vi "Brama_Sub_VI.vi"(6 "Enum in":T1(ring), 7 "Brama 1 - kto pierwszy":T5(ring), 9 "Brama 1":T4, 10 "reference in":refnum<vi>, 11 "Digital in":refnum<vi>) -> (2 "Enum out":T1(ring), 3 "Brama 2":T3)   [LabVIEW 2017]
uses:
  Str_Lam&Sil.ctl
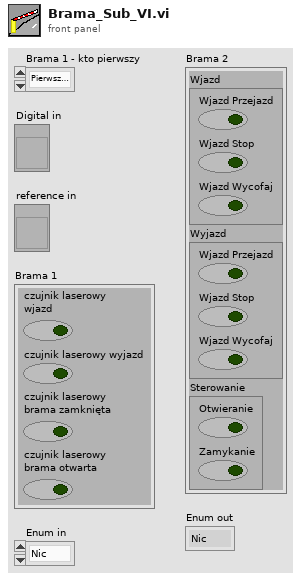
[diagram p1: front panel]
types:
  T1 = enum16{"Nic", "Otwieranie", "Otwarte", "Wjazd", "Wyjazd", "Zamykanie", "Wycofaj", "Blad"}
  T2 = typedef "Str_Lam&Sil.ctl" = bool
  T3 = cluster{"Wjazd":cluster{"Wjazd Przejazd":T2, "Wjazd Stop":bool, "Wjazd Wycofaj":bool}, "Wyjazd":cluster{"Wjazd Przejazd":bool, "Wjazd Stop":bool, "Wjazd Wycofaj":bool}, "Sterowanie":cluster{"Otwieranie":bool, "Zamykanie":bool}}
  T4 = cluster{"czujnik laserowy \nwjazd":bool, "czujnik laserowy wyjazd":bool, "czujnik laserowy \nbrama zamknięta":bool, "czujnik laserowy \nbrama otwarta":bool}
  T5 = enum16{"Pierwszy wjazd", "Nikt", "Pierwszy wyjazd"}
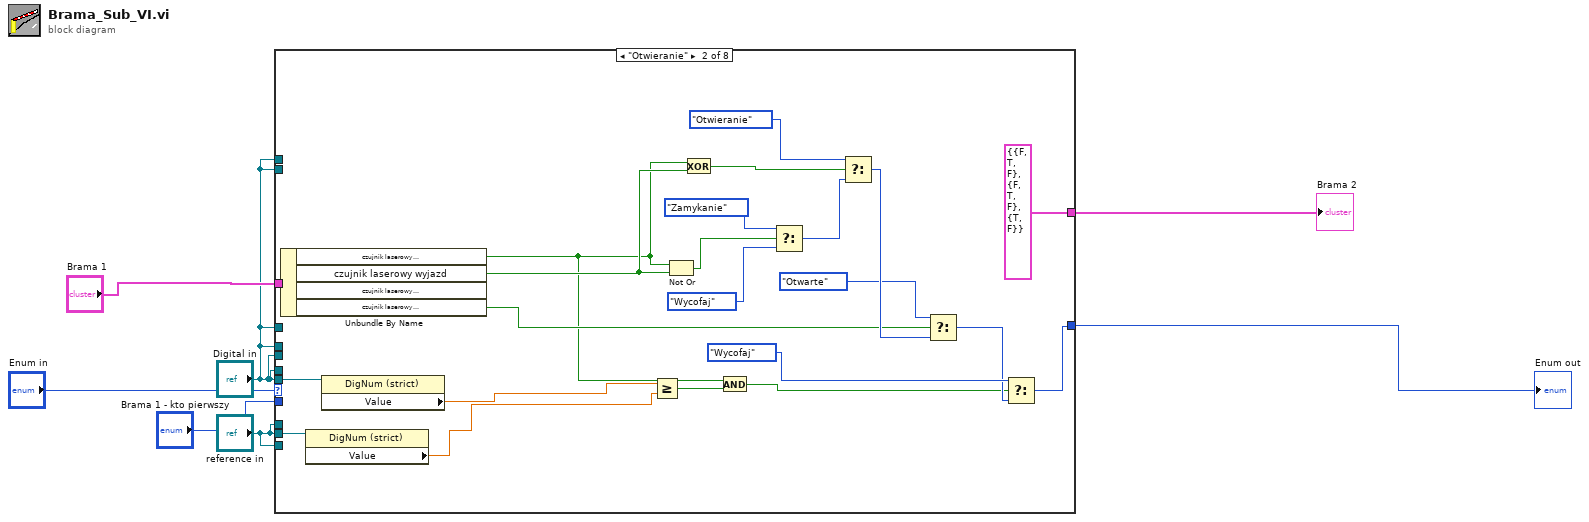
[diagram p0: block diagram]
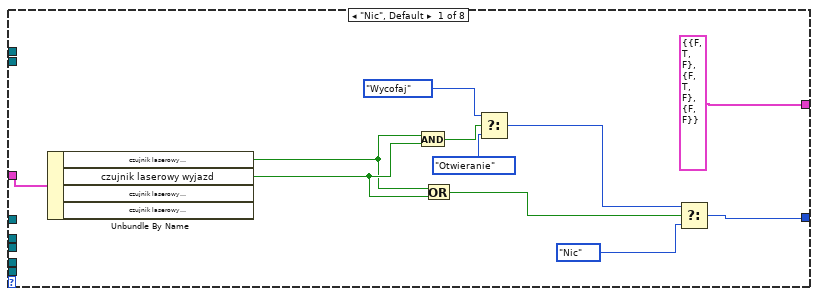
[diagram p2: hidden frame]
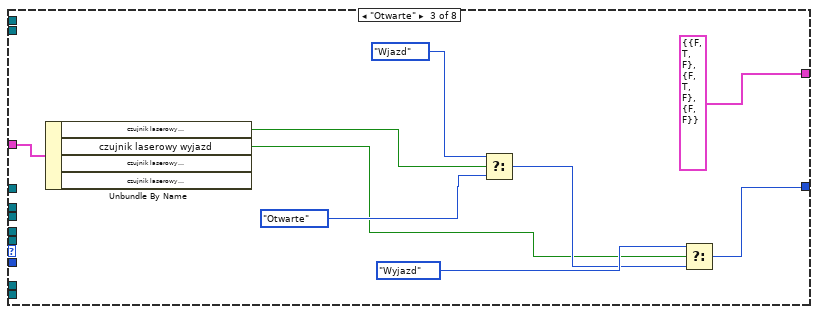
[diagram p3: hidden frame]
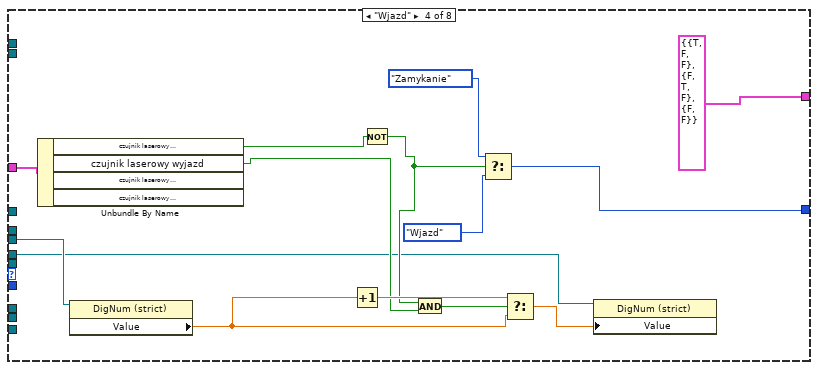
[diagram p4: hidden frame]
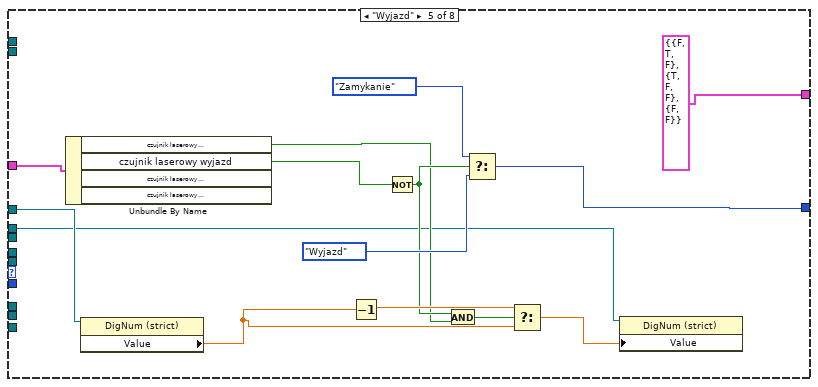
[diagram p5: hidden frame]
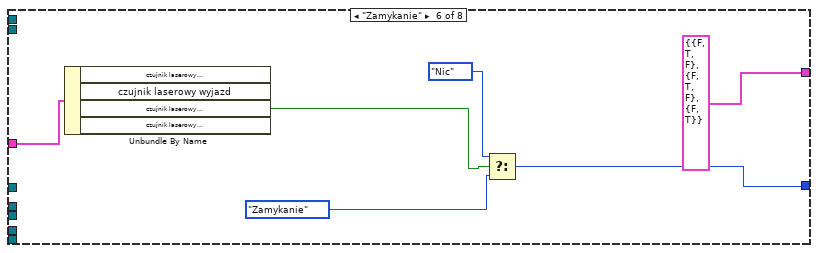
[diagram p6: hidden frame]
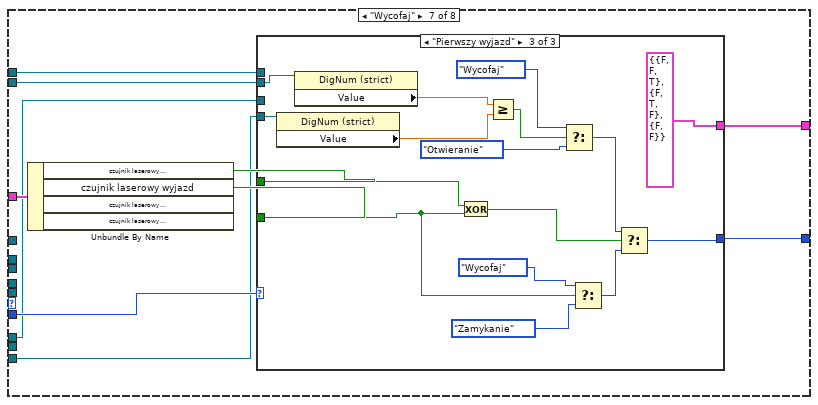
[diagram p7: hidden frame]
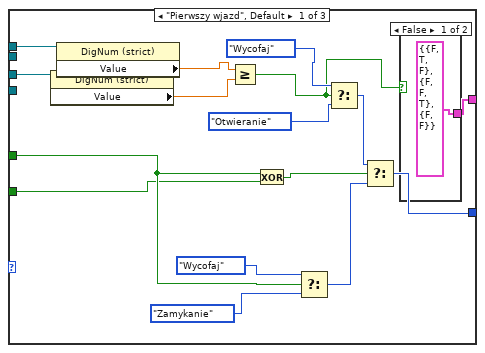
[diagram p8: hidden frame]
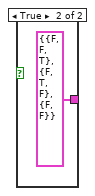
[diagram p9: hidden frame]
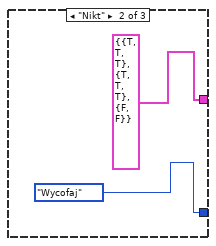
[diagram p10: hidden frame]
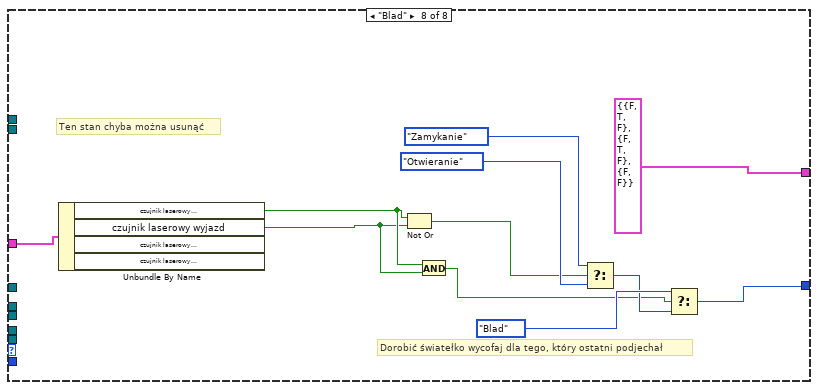
[diagram p11: hidden frame]
diagram:
  n1 = case shown="\"Otwieranie\"" "Enum in" {
    tunnel: "Brama 1" -> [w10 w40 w43 w61 w73 w80 w93 w139]
    tunnel: [w11 w27 w45 w60 w75 w78 w89 w136] -> w3
    tunnel: [T3 {"Wjazd"={"Wjazd Przejazd"=FALSE, "Wjazd Stop"=TRUE, "Wjazd Wycofaj"=FALSE}, "Wyjazd"={"Wjazd Przejazd"=FALSE, "Wjazd Stop"=TRUE, "Wjazd Wycofaj"=FALSE}, "Sterowanie"={"Otwieranie"=FALSE, "Zamykanie"=FALSE}} ("Brama 1") T3 {"Wjazd"={"Wjazd Przejazd"=FALSE, "Wjazd Stop"=TRUE, "Wjazd Wycofaj"=FALSE}, "Wyjazd"={"Wjazd Przejazd"=FALSE, "Wjazd Stop"=TRUE, "Wjazd Wycofaj"=FALSE}, "Sterowanie"={"Otwieranie"=TRUE, "Zamykanie"=FALSE}} ("Brama 1") T3 {"Wjazd"={"Wjazd Przejazd"=FALSE, "Wjazd Stop"=TRUE, "Wjazd Wycofaj"=FALSE}, "Wyjazd"={"Wjazd Przejazd"=FALSE, "Wjazd Stop"=TRUE, "Wjazd Wycofaj"=FALSE}, "Sterowanie"={"Otwieranie"=FALSE, "Zamykanie"=FALSE}} ("Brama 1") T3 {"Wjazd"={"Wjazd Przejazd"=TRUE, "Wjazd Stop"=FALSE, "Wjazd Wycofaj"=FALSE}, "Wyjazd"={"Wjazd Przejazd"=FALSE, "Wjazd Stop"=TRUE, "Wjazd Wycofaj"=FALSE}, "Sterowanie"={"Otwieranie"=FALSE, "Zamykanie"=FALSE}} ("Brama 1") T3 {"Wjazd"={"Wjazd Przejazd"=FALSE, "Wjazd Stop"=TRUE, "Wjazd Wycofaj"=FALSE}, "Wyjazd"={"Wjazd Przejazd"=TRUE, "Wjazd Stop"=FALSE, "Wjazd Wycofaj"=FALSE}, "Sterowanie"={"Otwieranie"=FALSE, "Zamykanie"=FALSE}} ("Brama 1") T3 {"Wjazd"={"Wjazd Przejazd"=FALSE, "Wjazd Stop"=TRUE, "Wjazd Wycofaj"=FALSE}, "Wyjazd"={"Wjazd Przejazd"=FALSE, "Wjazd Stop"=TRUE, "Wjazd Wycofaj"=FALSE}, "Sterowanie"={"Otwieranie"=FALSE, "Zamykanie"=TRUE}} ("Brama 1") w90 T3 {"Wjazd"={"Wjazd Przejazd"=FALSE, "Wjazd Stop"=TRUE, "Wjazd Wycofaj"=FALSE}, "Wyjazd"={"Wjazd Przejazd"=FALSE, "Wjazd Stop"=TRUE, "Wjazd Wycofaj"=FALSE}, "Sterowanie"={"Otwieranie"=FALSE, "Zamykanie"=FALSE}} ("Brama 1")] -> w4
    tunnel: "Brama 1 - kto pierwszy" -> [_ _ _ _ _ _ w88 _]
    tunnel: "Digital in" -> [_ w21 _ _ _ _ _ _]
    tunnel: "reference in" -> [_ w20 _ _ _ _ _ _]
    tunnel: "Digital in" -> [_ _ _ w51 _ _ _ _]
    tunnel: "Digital in" -> [_ _ _ w50 _ _ _ _]
    tunnel: "Digital in" -> [_ _ _ _ w65 _ _ _]
    tunnel: "Digital in" -> [_ _ _ _ w64 _ _ _]
    tunnel: "Digital in" -> [_ _ _ _ _ _ w87 _]
    tunnel: "reference in" -> [_ _ _ _ _ _ w86 _]
    tunnel: "Digital in" -> [_ _ _ _ _ _ w85 _]
    tunnel: "reference in" -> [_ _ _ _ _ _ w84 _]
    frame "Nic", Default {
      n2 = Unbundle By Name(w10) -> ("czujnik laserowy \nwjazd"=w8:bool, "czujnik laserowy wyjazd"=w16:bool)  [unwired: 2 out]
      n3 = And(x=w8, y=w16) -> (x .and. y?=w18:bool)
      n4 = Or(x=w8, y=w16) -> (x .or. y?=w15:bool)
      n5 = Select(t=T1."Wycofaj", s=w18, f=T1."Otwieranie") -> (s? t:f=w14:T1)
      n6 = Select(t=w14, s=w15, f=T1."Nic") -> (s? t:f=w11:T1)
    }
    frame "Otwieranie" {
      n7 = Unbundle By Name(w40) -> ("czujnik laserowy \nwjazd"=w24:bool, "czujnik laserowy wyjazd"=w31:bool, "czujnik laserowy \nbrama otwarta"=w37:bool)  [unwired: 1 out]
      n8 = property class="DigNum (strict)"(reference=w20) -> ("Value"=w23:dbl)  [unwired: 1 in, 2 out]
      n9 = property class="DigNum (strict)"(reference=w21) -> ("Value"=w22:dbl)  [unwired: 1 in, 2 out]
      n10 = Greater Or Equal?(x=w22, y=w23) -> (x >= y?=w25:bool)
      n11 = Not Or(1:w31, 2:w24) -> (0:w35:bool)
      n12 = Exclusive Or(1:w31, 2:w24) -> (0:w32:bool)
      n13 = And(x=w24, y=w25) -> (x .and. y?=w19:bool)
      n14 = Select(t=T1."Zamykanie", s=w35, f=T1."Wycofaj") -> (s? t:f=w29:T1)
      n15 = Select(t=T1."Otwieranie", s=w32, f=w29) -> (s? t:f=w38:T1)
      n16 = Select(t=T1."Otwarte", s=w37, f=w38) -> (s? t:f=w26:T1)
      n17 = Select(t=T1."Wycofaj", s=w19, f=w26) -> (s? t:f=w27:T1)
    }
    frame "Otwarte" {
      n18 = Unbundle By Name(w43) -> ("czujnik laserowy \nwjazd"=w42:bool, "czujnik laserowy wyjazd"=w41:bool)  [unwired: 2 out]
      n19 = Select(t=T1."Wjazd", s=w42, f=T1."Otwarte") -> (s? t:f=w46:T1)
      n20 = Select(t=T1."Wyjazd", s=w41, f=w46) -> (s? t:f=w45:T1)
    }
    frame "Wjazd" {
      n21 = Unbundle By Name(w61) -> ("czujnik laserowy \nwjazd"=w58:bool, "czujnik laserowy wyjazd"=w52:bool)  [unwired: 2 out]
      n22 = property class="DigNum (strict)"(reference=w51) -> ("Value"=w56:dbl)  [unwired: 1 in, 2 out]
      n23 = Increment(x=w56) -> (x+1=w57:dbl)
      n24 = Not(x=w58) -> (.not. x?=w53:bool)
      n25 = And(x=w53, y=w52) -> (x .and. y?=w54:bool)
      n26 = Select(t=T1."Zamykanie", s=w53, f=T1."Wjazd") -> (s? t:f=w60:T1)
      n27 = Select(t=w57, s=w54, f=w56) -> (s? t:f=w55:dbl)
      n28 = property class="DigNum (strict)"(reference=w50, "Value"=w55) -> ()  [unwired: 1 in, 2 out]
    }
    frame "Wyjazd" {
      n29 = Unbundle By Name(w73) -> ("czujnik laserowy \nwjazd"=w66:bool, "czujnik laserowy wyjazd"=w72:bool)  [unwired: 2 out]
      n30 = property class="DigNum (strict)"(reference=w65) -> ("Value"=w70:dbl)  [unwired: 1 in, 2 out]
      n31 = Decrement(x=w70) -> (x-1=w71:dbl)
      n32 = Not(x=w72) -> (.not. x?=w67:bool)
      n33 = And(x=w67, y=w66) -> (x .and. y?=w68:bool)
      n34 = Select(t=T1."Zamykanie", s=w67, f=T1."Wyjazd") -> (s? t:f=w75:T1)
      n35 = Select(t=w71, s=w68, f=w70) -> (s? t:f=w69:dbl)
      n36 = property class="DigNum (strict)"(reference=w64, "Value"=w69) -> ()  [unwired: 1 in, 2 out]
    }
    frame "Zamykanie" {
      n37 = Unbundle By Name(w80) -> ("czujnik laserowy \nbrama zamknięta"=w79:bool)  [unwired: 3 out]
      n38 = Select(t=T1."Nic", s=w79, f=T1."Zamykanie") -> (s? t:f=w78:T1)
    }
    frame "Wycofaj" {
      n39 = Unbundle By Name(w93) -> ("czujnik laserowy \nwjazd"=w91:bool, "czujnik laserowy wyjazd"=w92:bool)  [unwired: 2 out]
      n40 = case shown="\"Pierwszy wjazd\", Default" w88 {
        tunnel: w92 -> [w103 _ w122]
        tunnel: w91 -> [w104 _ w127]
        tunnel: [w97 T3 {"Wjazd"={"Wjazd Przejazd"=TRUE, "Wjazd Stop"=TRUE, "Wjazd Wycofaj"=TRUE}, "Wyjazd"={"Wjazd Przejazd"=TRUE, "Wjazd Stop"=TRUE, "Wjazd Wycofaj"=TRUE}, "Sterowanie"={"Otwieranie"=FALSE, "Zamykanie"=FALSE}} ("Brama 1") T3 {"Wjazd"={"Wjazd Przejazd"=FALSE, "Wjazd Stop"=FALSE, "Wjazd Wycofaj"=TRUE}, "Wyjazd"={"Wjazd Przejazd"=FALSE, "Wjazd Stop"=TRUE, "Wjazd Wycofaj"=FALSE}, "Sterowanie"={"Otwieranie"=FALSE, "Zamykanie"=FALSE}} ("Brama 1")] -> w90
        tunnel: [w109 T1."Wycofaj" w128] -> w89
        tunnel: w87 -> [w95 _ _]
        tunnel: w86 -> [w94 _ _]
        tunnel: w85 -> [_ _ w115]
        tunnel: w84 -> [_ _ w114]
        frame "Pierwszy wjazd", Default {
          n41 = property class="DigNum (strict)"(reference=w94) -> ("Value"=w101:dbl)  [unwired: 1 in, 2 out]
          n42 = property class="DigNum (strict)"(reference=w95) -> ("Value"=w102:dbl)  [unwired: 1 in, 2 out]
          n43 = Greater Or Equal?(x=w102, y=w101) -> (x >= y?=w96:bool)
          n44 = Exclusive Or(1:w103, 2:w104) -> (0:w105:bool)
          n45 = Select(t=T1."Wycofaj", s=w104, f=T1."Zamykanie") -> (s? t:f=w106:T1)
          n46 = Select(t=T1."Wycofaj", s=w96, f=T1."Otwieranie") -> (s? t:f=w98:T1)
          n47 = Select(t=w98, s=w105, f=w106) -> (s? t:f=w109:T1)
          n48 = case shown="False" w96 {
            tunnel: [T3 {"Wjazd"={"Wjazd Przejazd"=FALSE, "Wjazd Stop"=TRUE, "Wjazd Wycofaj"=FALSE}, "Wyjazd"={"Wjazd Przejazd"=FALSE, "Wjazd Stop"=FALSE, "Wjazd Wycofaj"=TRUE}, "Sterowanie"={"Otwieranie"=FALSE, "Zamykanie"=FALSE}} ("Brama 1") T3 {"Wjazd"={"Wjazd Przejazd"=FALSE, "Wjazd Stop"=FALSE, "Wjazd Wycofaj"=TRUE}, "Wyjazd"={"Wjazd Przejazd"=FALSE, "Wjazd Stop"=TRUE, "Wjazd Wycofaj"=FALSE}, "Sterowanie"={"Otwieranie"=FALSE, "Zamykanie"=FALSE}} ("Brama 1")] -> w97
            frame False {
            }
            frame True {
            }
          }
        }
        frame "Nikt" {
        }
        frame "Pierwszy wyjazd" {
          n49 = property class="DigNum (strict)"(reference=w114) -> ("Value"=w118:dbl)  [unwired: 1 in, 2 out]
          n50 = property class="DigNum (strict)"(reference=w115) -> ("Value"=w117:dbl)  [unwired: 1 in, 2 out]
          n51 = Exclusive Or(1:w122, 2:w127) -> (0:w126:bool)
          n52 = Greater Or Equal?(x=w117, y=w118) -> (x >= y?=w116:bool)
          n53 = Select(t=T1."Wycofaj", s=w116, f=T1."Otwieranie") -> (s? t:f=w120:T1)
          n54 = Select(t=T1."Wycofaj", s=w122, f=T1."Zamykanie") -> (s? t:f=w123:T1)
          n55 = Select(t=w120, s=w126, f=w123) -> (s? t:f=w128:T1)
        }
      }
    }
    frame "Blad" {
      # "Ten stan chyba można usunąć"
      # "Dorobić światełko wycofaj dla tego, który ostatni podjechał"
      n56 = Unbundle By Name(w139) -> ("czujnik laserowy \nwjazd"=w132:bool, "czujnik laserowy wyjazd"=w131:bool)  [unwired: 2 out]
      n57 = Not Or(1:w131, 2:w132) -> (0:w133:bool)
      n58 = And(x=w132, y=w131) -> (x .and. y?=w130:bool)
      n59 = Select(t=T1."Zamykanie", s=w133, f=T1."Otwieranie") -> (s? t:f=w134:T1)
      n60 = Select(t=T1."Blad", s=w130, f=w134) -> (s? t:f=w136:T1)
    }
  }
  "Brama 2" <- w4
  "Enum out" <- w3
